vi "Switch magnet  fc open.vi"(0 "Faraday cup":bool) -> ()   [LabVIEW 2012]
doc: "This vi will raise and lower faraday cups that use switches"
panel:
  out "error out":errorcluster
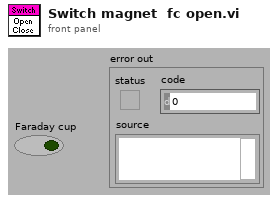
[diagram p1: front panel]
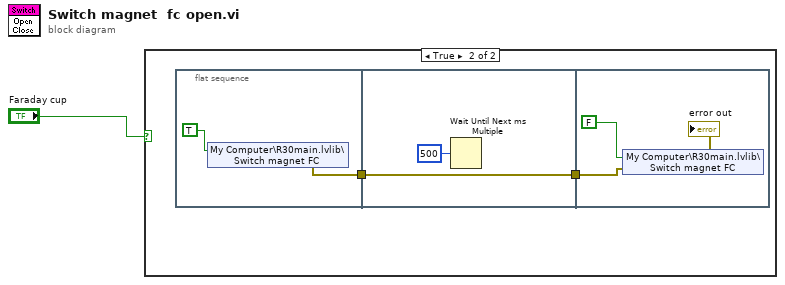
[diagram p0: block diagram]
diagram:
  n1 = case shown="True" "Faraday cup" {
    frame False {
    }
    frame True {
      n2 = flat-sequence {
        tunnel: [w4] -> w2
        tunnel: [w6] -> w3
        tunnel: w2 -> [w6]
        tunnel: w3 -> [w9]
        frame #0 {
          n3 = shared-variable "My Computer\\R30main.lvlib\\Switch magnet FC"(TRUE ("INJ Image FC")) -> (error out=w4:errorcluster)  [unwired: 1 out]
        }
        frame #1 {
          n4 = Wait Until Next ms Multiple(millisecond multiple=u32 500) -> ()  [unwired: 1 out]
        }
        frame #2 {
          n5 = shared-variable "My Computer\\R30main.lvlib\\Switch magnet FC"(FALSE ("INJ Image FC"), error in=w9) -> (error out=→"error out":errorcluster)
        }
      }
    }
  }
